vi "Programmatic API Tree.vi"   [LabVIEW 2011, in "VI Tester API.lvlib"]
doc: "Programmatic API VIs for VI Tester"
uses:
  VI Tester API.lvlib
  Classes/TestCase/TestCase.lvclass
  Classes/TestSuite/TestSuite.lvclass
panel:
  # "JKI VI Tester for LabVIEW\nhttp://jkisoft.com/vi-tester\nCopyright (C) 2007-2009, JKI <info@jkisoft.com>\nALL RIGHTS RESERVED"
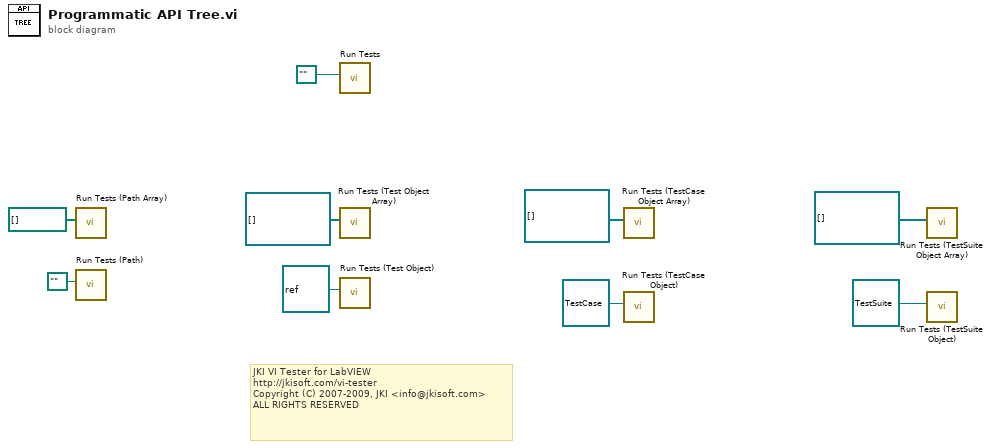
[diagram p0: block diagram]
diagram:
  # "JKI VI Tester for LabVIEW\nhttp://jkisoft.com/vi-tester\nCopyright (C) 2007-2009, JKI <info@jkisoft.com>\nALL RIGHTS RESERVED"
  n1 = call "Run Tests (Path Array).vi"("Test Paths"=path[] []) -> ()  [unwired: 8 in, 3 out]
  n2 = call "Run Tests (Path).vi"("Test Path"=path "") -> ()  [unwired: 8 in, 3 out]
  n3 = call-poly "Run Tests.vi"("Test Path"=path "" ("Project")) -> ()  [unwired: 8 in, 3 out]
  n4 = call "Run Tests (Test Object Array).vi"("Tests"=refnum<class>[] []) -> ()  [unwired: 8 in, 3 out]
  n5 = call "Run Tests (Test Object).vi"("Test"=refnum<class> refnum) -> ()  [unwired: 8 in, 3 out]
  n6 = call "Run Tests (TestCase Object Array).vi"("TestCase Objects"=refnum<class "TestCase.lvclass">[] []) -> ()  [unwired: 8 in, 3 out]
  n7 = call "Run Tests (TestCase Object).vi"("TestCase"=refnum<class "TestCase.lvclass"> refnum) -> ()  [unwired: 8 in, 3 out]
  n8 = call "Run Tests (TestSuite Object Array).vi"("TestCase Objects"=refnum<class "TestSuite.lvclass">[] []) -> ()  [unwired: 8 in, 3 out]
  n9 = call "Run Tests (TestSuite Object).vi"("TestSuite"=refnum<class "TestSuite.lvclass"> refnum) -> ()  [unwired: 8 in, 3 out]
